vi "XYStage.GetPrivateEventsRegistration.vi"(8 "error in (no error)":errorcluster, 11 "XYStage in":refnum<class "XYStage.lvclass">) -> (0 "error out":errorcluster, 2 "XYStage Private Events":refnum<event-registration>, 3 "XYStage out":refnum<class "XYStage.lvclass">)   [LabVIEW 2017, in "XYStage.lvclass"]
uses:
  XYStage.lvclass
  Typedefs/PrivateEvents--Cluster.ctl
  Typedefs/PrivateEvents--XYStage.MoveAbsolute (units).ctl
  Typedefs/Coordinates.Units--Cluster.ctl
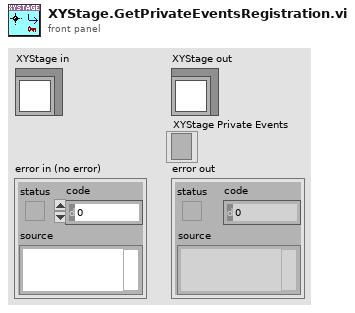
[diagram p1: front panel]
types:
  T1 = typedef "XYStage.lvclass/PrivateEvents--Cluster.ctl" = cluster{"MoveAbsolute (units)":refnum<user-event>}
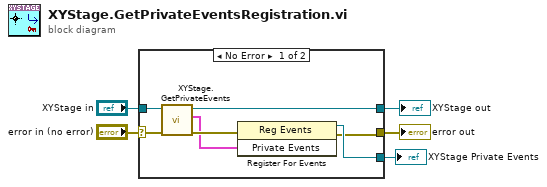
[diagram p0: block diagram]
diagram:
  n1 = case shown="No Error" "error in (no error)" {
    selector: "error in (no error)" -> [w11 w14]
    tunnel: [w6 w14] -> w4
    tunnel: [w10 w13] -> w2
    tunnel: "XYStage in" -> [w12 w13]
    tunnel: [w7 _] -> w1
    frame No Error {
      n2 = call "XYStage.GetPrivateEvents.vi"("error in (no error)"=w11, "XYStage"=w12) -> ("error out"=w9:errorcluster, "Private Events"=w8:T1, "XYStage out"=w10:refnum<class "XYStage.lvclass">)  [unwired: 7 in]
      n3 = register-events(error in=w9, w8) -> (reference out=w7:refnum<event-registration>, error out=w6:errorcluster)  [unwired: 1 in]
    }
    frame Error {
    }
  }
  "error out" <- w4
  "XYStage out" <- w2
  "XYStage Private Events" <- w1
